vi "json.generate_object.vi"(8 "error in":errorcluster, 11 "ts.relative in":refnum<class "ts.relative.lvclass">) -> (0 "error out":errorcluster, 2 "JSON Object":string, 3 "ts.relative out":refnum<class "ts.relative.lvclass">)   [LabVIEW 2020, in "ts.relative.lvclass"]
uses:
  ts.relative.lvclass
  C:/code/labview-client/lv_src/timestampMetadata/timestampMetadata.lvclass
  ts.relative.lvclass/ts.relative.ctl
  timestampMetadata/timestampMetadata.lvclass/timestampMetadata.ctl
  58b5a3bf-67b0-4cfc-be86-d8802f060b17.vi
  0a5a6386-9c4a-4c3b-8002-10d1d06bec1e.vi
  timestampMetadata/seriesName.get.vi
  <vilib>/JDP Science/JSONtext/Variant to JSON Text.vi
  <vilib>/LabVIEW Open Source Project/Epoch Date & Time/formatter.iso8601/Timestamp to ISO8601 UTC DateTime.vi
  <vilib>/JDP Science/JSONtext/LVClass Serializer/JSONtext LVClass Serializer.lvclass
  Nominal Client/Nominal Client.lvclass
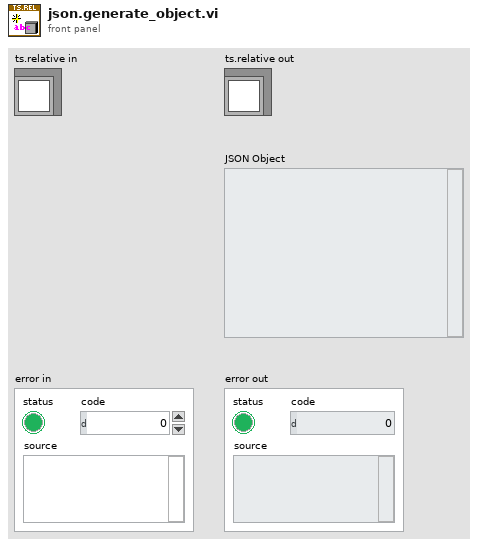
[diagram p1: front panel]
types:
  T1 = enum16{"DAYS", "HOURS", "MINUTES", "SECONDS", "MILLISECONDS", "MICROSECONDS", "NANOSECONDS", "PICOSECONDS"}
  T2 = cluster{"seriesName":string, "timestampType":cluster{"type":string, "relative":cluster{"timeUnit":string}}}
  T3 = cluster{"seriesName":string, "timestampType":cluster{"type":string, "relative":cluster{"timeUnit":string, "offset":string}}}
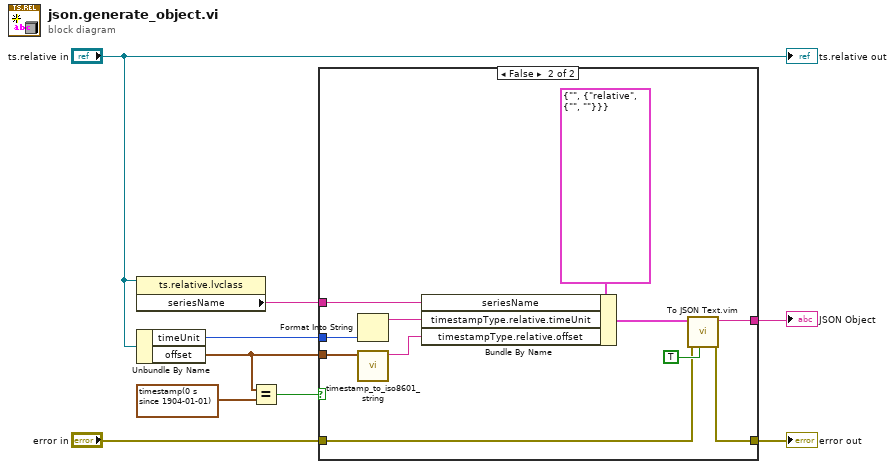
[diagram p0: block diagram]
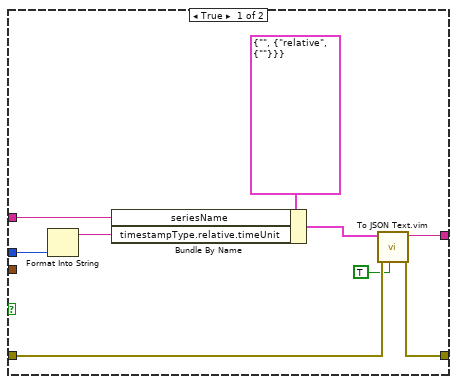
[diagram p2: hidden frame]
diagram:
  n1 = property class="ts.relative.lvclass"(reference="ts.relative in") -> ("seriesName"=w8:string)  [unwired: 1 in, 2 out]
  n2 = Unbundle By Name("ts.relative in") -> ("timeUnit"=w7:T1, "offset"=w6:timestamp)
  n3 = Equal?(x=w6, y=timestamp(0 s since 1904-01-01) ("offset")) -> (x = y?=w1:bool)
  n4 = case shown="False" w1 {
    tunnel: w8 -> [w17 w28]
    tunnel: w7 -> [w16 w27]
    tunnel: w6 -> [_ w20]
    tunnel: [w13 w24] -> w4
    tunnel: [w12 w22] -> w3
    tunnel: "error in" -> [w11 w21]
    frame True {
      n5 = Format Into String(w16) -> (resulting string=w15:string)  [unwired: 3 in, 1 out]
      n6 = Bundle By Name(cluster=T2 {"seriesName"="", "timestampType"={"type"="relative", "relative"={"timeUnit"=""}}}, "seriesName"=w17, "timestampType.relative.timeUnit"=w15) -> (w14:T2)
      n7 = call "To JSON Text.vim"("Pretty Print?"=TRUE, "error in (no error)"=w11, "Anything"=w14) -> ("error out"=w12:errorcluster, "<JSON>"=w13:string)  [unwired: 7 in]
    }
    frame False {
      n8 = Format Into String(w27) -> (resulting string=w26:string)  [unwired: 3 in, 1 out]
      n9 = call "timestamp_to_iso8601_string.vi"("Time Stamp (now)"=w20) -> ("ISO8601 UTC DateTime"=w19:string)  [unwired: 10 in]
      n10 = Bundle By Name(cluster=T3 {"seriesName"="", "timestampType"={"type"="relative", "relative"={"timeUnit"="", "offset"=""}}}, "seriesName"=w28, "timestampType.relative.timeUnit"=w26, "timestampType.relative.offset"=w19) -> (w25:T3)
      n11 = call "To JSON Text.vim"("Pretty Print?"=TRUE, "error in (no error)"=w21, "Anything"=w25) -> ("error out"=w22:errorcluster, "<JSON>"=w24:string)  [unwired: 7 in]
    }
  }
  "error out" <- w3
  "JSON Object" <- w4
  "ts.relative out" <- "ts.relative in"
